vi "TestExec.Process Options for Archive UUT Folder.vi"(6 "Sequence":string, 7 "Code":string, 8 "Result":string, 9 "Args":string[](array[string]), 10 "ArchiveDir":path, 11 "UUTDir":path) -> (0 "Error":errorcluster, 1 "SubDirs":string[](array[string]), 2 "New Name":string, 3 "Destination Path":path)   [LabVIEW 2018]
panel:
  # "AppendSeq, AppendResult, $Date, $Mode"
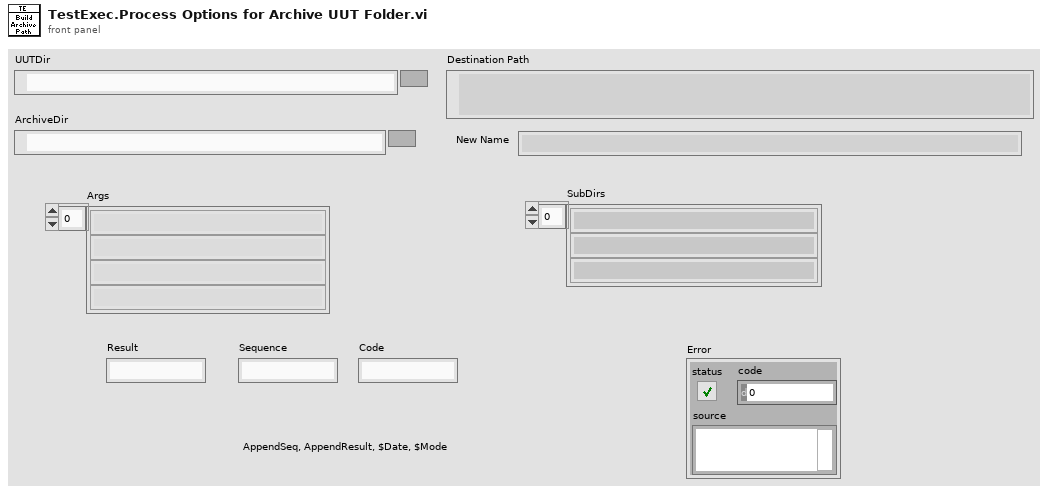
[diagram p1: front panel]
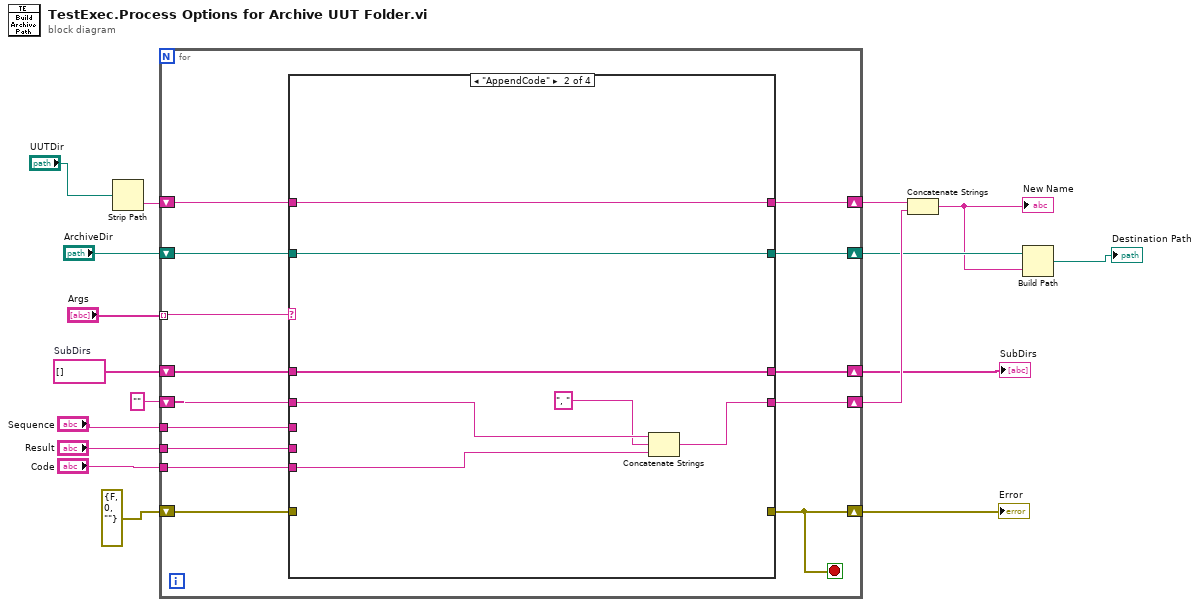
[diagram p0: block diagram]
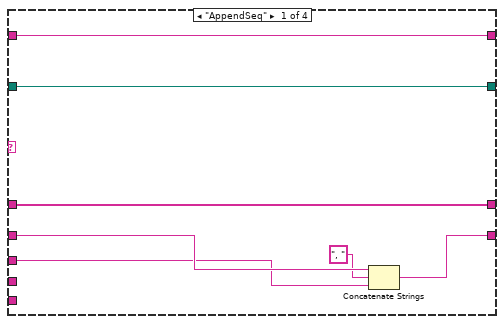
[diagram p2: hidden frame]
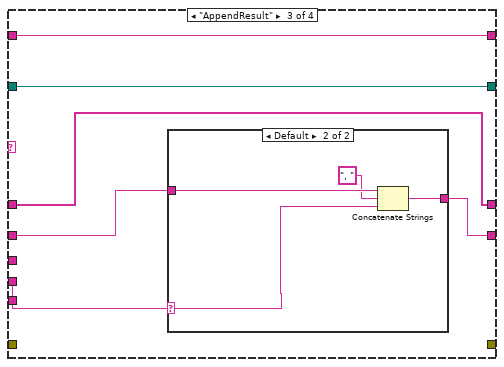
[diagram p3: hidden frame]
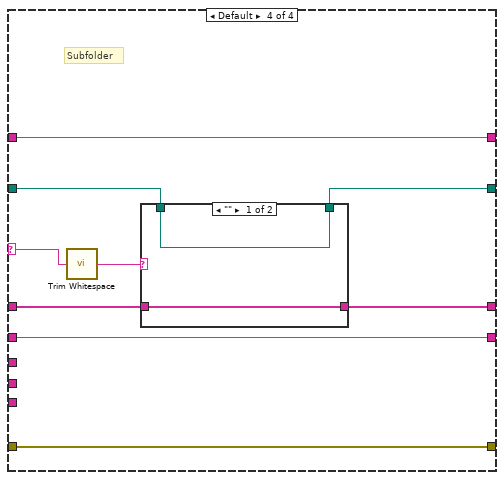
[diagram p5: hidden frame]
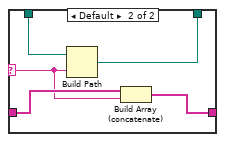
[diagram p6: hidden frame]
diagram:
  w3 = string[] []  # SubDirs
  n1 = Strip Path(path="UUTDir") -> (name=w11:string)  [unwired: 1 out]
  n2 = for {
    tunnel: "Args" -> [w21] mode=indexing
    shift-right: [w26] -> w9
    shift-left: "" -> [w29]
    shift-right: [w28] -> w10
    shift-left: w11 -> [w30]
    shift-right: [w27] -> w8
    shift-left: "ArchiveDir" -> [w31]
    tunnel: "Sequence" -> [w25]
    tunnel: "Result" -> [w24]
    shift-right: [w22] -> w5
    shift-left: errorcluster {"status"=FALSE, "code"=0, "source"=""} ("error constant") -> [w23]
    shift-right: [w19] -> w2
    shift-left: w3 -> [w20]
    tunnel: "Code" -> [w18]
    stop <- w22 stop-if-true
    n3 = case shown="\"AppendCode\"" w21 {
      selector: w21 -> [_ _ _ w61]
      tunnel: w31 -> [w36 w43 w49 w62]
      tunnel: w30 -> [w37 w44 w50 w65]
      tunnel: w29 -> [w38 w45 w51 w64]
      tunnel: [w37 w44 w50 w65] -> w28
      tunnel: [w36 w43 w49 w60] -> w27
      tunnel: [w35 w42 w48 w64] -> w26
      tunnel: w25 -> [w34 _ _ _]
      tunnel: w24 -> [_ _ w47 _]
      tunnel: w23 -> [_ _ _ w59]
      tunnel: [_ _ _ w59] -> w22
      tunnel: w20 -> [w32 w40 w46 w58]
      tunnel: [w32 w40 w46 w57] -> w19
      tunnel: w18 -> [_ w39 _ _]
      frame "AppendSeq" {
        n4 = Concatenate Strings(w38, ", ", w34) -> (w35:string)
      }
      frame "AppendCode" {
        n5 = Concatenate Strings(w45, ", ", w39) -> (w42:string)
      }
      frame "AppendResult" {
        n6 = case shown="Default" w47 {
          selector: w47 -> [_ w53]
          tunnel: w51 -> [w52 w56]
          tunnel: [w52 w55] -> w48
          frame "" {
            # "Do nothing"
          }
          frame Default {
            n7 = Concatenate Strings(w56, ", ", w53) -> (w55:string)
          }
        }
      }
      frame Default {
        # "Subfolder"
        n8 = call <vilib>:"Trim Whitespace.vi"("string"=w61) -> ("trimmed string"=w63:string)  [unwired: 1 in]
        n9 = case shown="\"\"" w63 {
          selector: w63 -> [_ w69]
          tunnel: w62 -> [w67 w72]
          tunnel: [w67 w71] -> w60
          tunnel: w58 -> [w66 w70]
          tunnel: [w66 w68] -> w57
          frame "" {
          }
          frame Default {
            n10 = Build Path(base path=w72, name or relative path=w69) -> (appended path=w71:path)
            n11 = Build Array (concatenate)(w70, w69) -> (w68:string[])
          }
        }
      }
    }
  }
  "Error" <- w5
  "SubDirs" <- w2
  n12 = Concatenate Strings(w10, w9) -> (w4:string)
  "New Name" <- w4
  n13 = Build Path(base path=w8, name or relative path=w4) -> (appended path=→"Destination Path":path)
